vi "set_params.vi"(8 "error in (no error)":errorcluster caption="entrée d'erreur (pas d'erreur)", 11 "SpectralCoclustering.lvclass 2":refnum<class "SpectralCoclustering.lvclass">) -> (0 "error out":errorcluster caption="sortie d'erreur", 3 "SpectralCoclustering.lvclass":refnum<class "SpectralCoclustering.lvclass">)   [LabVIEW 2020, in "SpectralCoclustering.lvclass"]
uses:
  SpectralCoclustering.lvclass
  SpectralCoclustering.lvclass/SpectralCoclustering.ctl
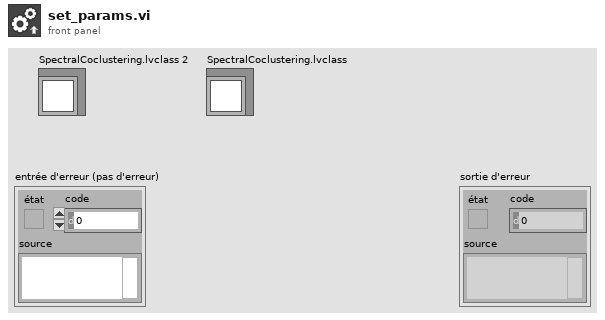
[diagram p1: front panel]
types:
  T1 = typedef "spectral_coclustering_params.ctl" = cluster{"n_clusters":dbl, "svd_method":string, "n_svd_vecs":cluster{"n_svd_vecs_type":string, "n_svd_int":dbl}, "mini_batch":bool, "init":cluster{"init_type":string, "init_list":dbl[][]}, "n_init":dbl, "random_state":dbl}
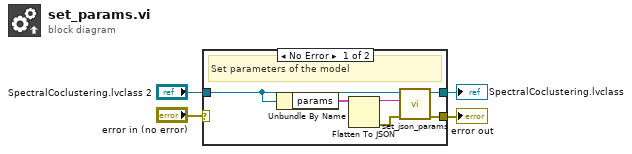
[diagram p0: block diagram]
diagram:
  n1 = case shown="No Error" "error in (no error)" {
    selector: "error in (no error)" -> [_ w12]
    tunnel: [w7 w12] -> w3
    tunnel: [w8 w11] -> w1
    tunnel: "SpectralCoclustering.lvclass 2" -> [w5 w11]
    frame No Error {
      # "Set parameters of the model"
      n2 = Unbundle By Name(w5) -> ("params"=w10:T1)
      n3 = Flatten To JSON(anything=w10) -> (JSON string=w9:string, 11:w6:errorcluster)  [unwired: 2 in]
      n4 = call-dynamic "set_json_params.vi"("error in (no error)"=w6, "params"=w9, "Model en entrée"=w5) -> ("error out"=w7:errorcluster, "Model en sortie"=w8:refnum<class "SpectralCoclustering.lvclass">)  [unwired: 7 in]
    }
    frame Error {
    }
  }
  "error out" <- w3
  "SpectralCoclustering.lvclass" <- w1
